vi "Insert Image (Greyscale).vi"(7 "Offset (Default: 0,0)":T1, 8 "error in (no error)":errorcluster, 9 "Greyscale Image Destination":T2, 10 "Greyscale Image Child":T2, 11 "Greyscale Image Parent":T2) -> (0 "error out":errorcluster, 3 "Greyscale Image Destination (duplicate)":T2)   [LabVIEW 2020, in "image.lvlib"]
uses:
  image.lvlib
  Greyscale Image.ctl
  common/Image Point (Integer).ctl
  5e3288c8-ee88-4cfe-89cf-31ceca475f5a.vi
  common/Module Path.vi
  <vilib>/Utility/error.llb/Error Cluster From Error Code.vi
  common/common.lvlib
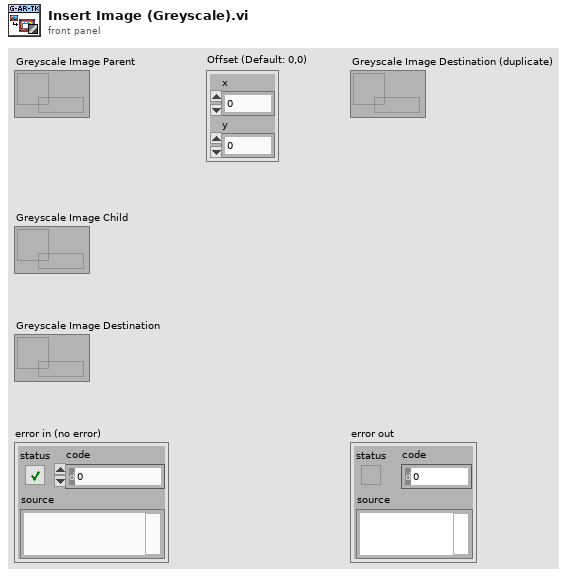
[diagram p1: front panel]
types:
  T1 = typedef "common.lvlib/Image Point (Integer).ctl" = cluster{"x":i32, "y":i32}
  T2 = typedef "image.lvlib/Greyscale Image.ctl" = refnum<data-value>
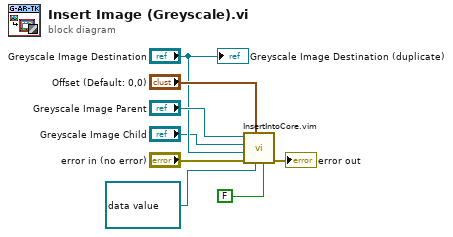
[diagram p0: block diagram]
diagram:
  n1 = call "InsertIntoCore.vim"("Has Mask"=FALSE, "Mask"=refnum<data-value> refnum, "Offset"="Offset (Default: 0,0)", "error in (no error)"="error in (no error)", "Dst"="Greyscale Image Destination", "Src_Child"="Greyscale Image Child", "Src_Parent"="Greyscale Image Parent") -> ("error out"=→"error out":errorcluster)  [unwired: 4 in]
  "Greyscale Image Destination (duplicate)" <- "Greyscale Image Destination"
